vi "RichToFlatcif_manager_LoaderInfoFull.vi"(5 "OutputClusterType":T1, 11 "InputCluster":T3) -> (3 "OutputCluster":T1)   [LabVIEW 2021, in "CIF_Manager_client.lvlib"]
uses:
  CIF_Manager_client.lvlib
  cif_manager_LoaderInfoFull.ctl
  cif_manager_LoaderType.ctl
  cif_manager_LoaderInfoFull_Flat.ctl
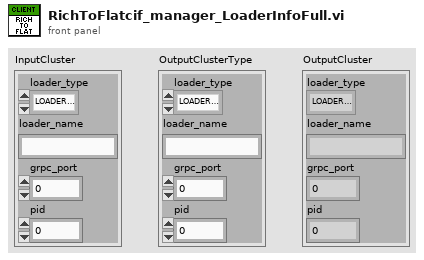
[diagram p1: front panel]
types:
  T1 = typedef "CIF_Manager_client.lvlib/cif_manager_LoaderInfoFull_Flat.ctl" = cluster{"loader_type":T2, "loader_name":string, "grpc_port":i32, "pid":u32}
  T2 = typedef "CIF_Manager_client.lvlib/cif_manager_LoaderType.ctl" = enum32{"LOADERTYPE_UNKNOWN", "LOADERTYPE_LABVIEW"}
  T3 = typedef "CIF_Manager_client.lvlib/cif_manager_LoaderInfoFull.ctl" = cluster{"loader_type":T2, "loader_name":string, "grpc_port":i32, "pid":u32}
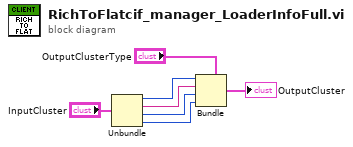
[diagram p0: block diagram]
diagram:
  n1 = Unbundle "Unbundle"("InputCluster") -> ("loader_type"=w4:T2, "loader_name"=w3:string, "grpc_port"=w2:i32, "pid"=w1:u32)
  n2 = Bundle "Bundle"(cluster="OutputClusterType", "loader_type"=w4, "loader_name"=w3, "grpc_port"=w2, "pid"=w1) -> (→"OutputCluster":T1)
